vi "Update Vehicle Position.vi"(8 "error in (no error)":errorcluster, 10 "Vehicle Position":T1, 11 "Vehicle Position Interface Simulation in":refnum<class "Vehicle Position Interface Simulation.lvclass">) -> (0 "error out":errorcluster, 3 "Vehicle Position Interface Simulation out":refnum<class "Vehicle Position Interface Simulation.lvclass">)   [LabVIEW 2012, in "Vehical Position Interface Simulation.lvlib" / "Vehicle Position Interface Simulation.lvclass"]
uses:
  Vehicle Position Interface Simulation.lvclass
  Car Wash Controller/Car Wash Controller/Vehicle Position.ctl
  Vehical Position Interface API/Vehical Position Interface API/Vehicle Position Interface API.lvclass
  Car Wash Controller/Car Wash Controller/Car Wash Controller.lvclass
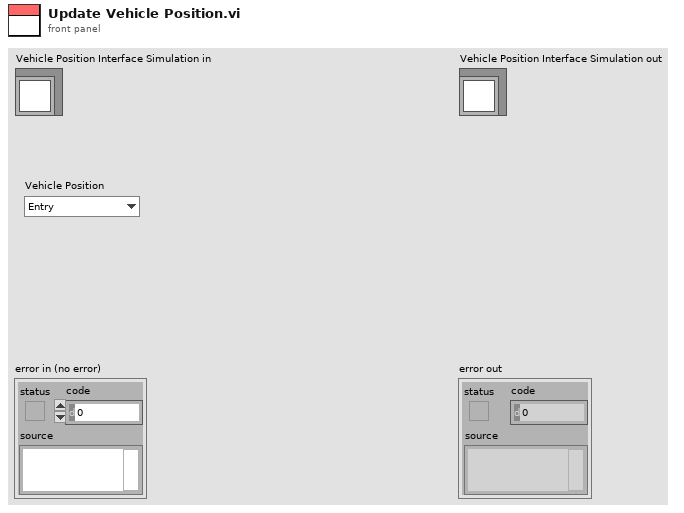
[diagram p1: front panel]
types:
  T1 = typedef "Car Wash Controller.lvlib/Car Wash Controller.lvclass/Vehicle Position.ctl" = enum16{"Entry", "Station 1", "Station 2", "Station 3", "Exit"}
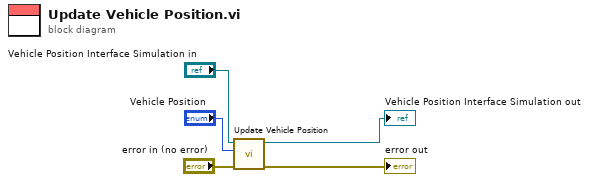
[diagram p0: block diagram]
diagram:
  n1 = call-parent "Update Vehicle Position.vi"("error in (no error)"="error in (no error)", "Vehicle Position"="Vehicle Position", "Vehicle Position Interface API in"="Vehicle Position Interface Simulation in") -> ("error out"=→"error out":errorcluster, "Vehicle Position Interface API out"=→"Vehicle Position Interface Simulation out":refnum<class "Vehicle Position Interface Simulation.lvclass">)  [unwired: 7 in]
